vi "2 - Use the NI-DAQmx VIs (Original).vi"() -> ()   [LabVIEW 2012]
uses:
  <vilib>/DAQmx/read.llb/DAQmx Read (Analog 1D Wfm NChan NSamp).vi
  <vilib>/DAQmx/create/channels.llb/DAQmx Create Channel (AI-Temperature-Thermocouple).vi
  <resource>/objmgr/daqmx.rc
panel:
  out "Alarm Output":bool
  in  "Alarm Level":dbl=26.0
  out "Temperature":waveform(dbl)[](graph)
  in  "stop":bool
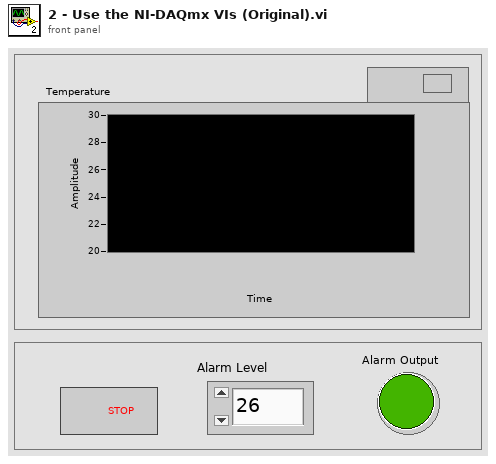
[diagram p1: front panel]
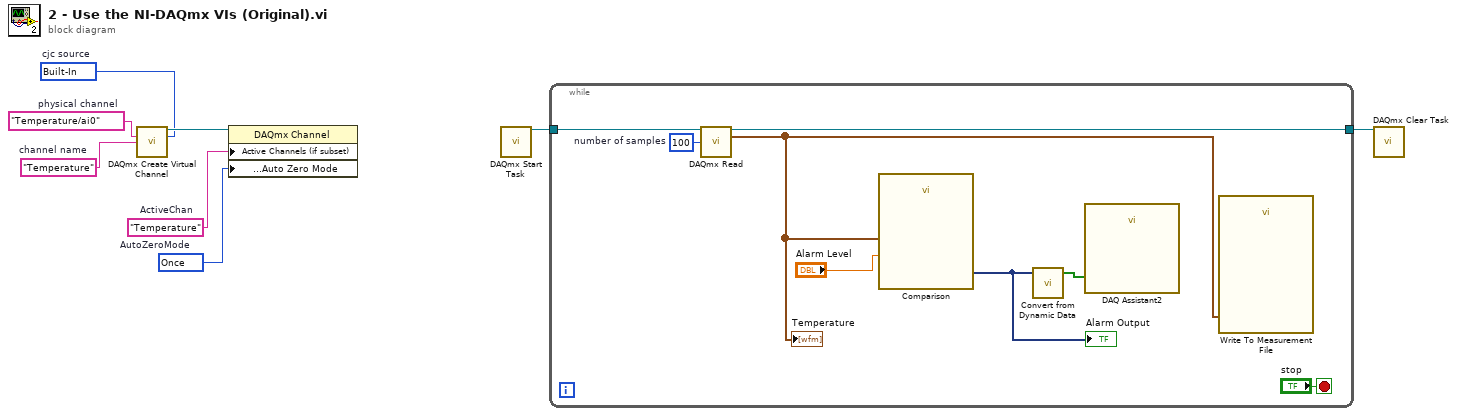
[diagram p0: block diagram]
diagram:
  w1 = tag "Temperature/ai0"  # physical channel
  w3 = 10200 items=["Built-In"=10200, "Constant Value"=10116, "Channel"=10113]  # cjc source
  w2 = 10244 items=["None"=10230, "Once"=10244, "Every Sample"=10164]  # AutoZeroMode
  w4 = "Temperature"  # ActiveChan
  w6 = "Temperature"  # channel name
  n1 = call-poly <vilib>:"DAQmx Create Virtual Channel.vi"("physical channels"=w1, "cjc source"=w3, "name to assign"=w6) -> ("task out"=w5:refnum<k21>)  [unwired: 11 in, 1 out]
  n2 = property class="DAQmx Channel"(reference=w5, "Active Channels (if subset)"=w4, "Analog Input:General Properties:Advanced:High Accuracy Settings:Auto Zero Mode"=w2) -> ()  [unwired: 1 in, 2 out]
  n3 = call <vilib>:"DAQmx Start Task.vi"() -> ("task out"=w8:refnum<k21>)  [unwired: 14 in, 1 out]
  n4 = while {
    tunnel: w8 -> [w12]
    tunnel: [w11] -> w7
    stop <- "stop" stop-if-true
    w9 = 100  # number of samples
    n5 = call-poly <vilib>:"DAQmx Read.vi"("task/channels in"=w12, "number of samples per channel"=w9) -> ("task out"=w11:refnum<k21>, "data"=w10:waveform(dbl)[])  [unwired: 11 in, 1 out]
    "Temperature" <- w10
    n6 = call "Comparison"("Operand 2"="Alarm Level", "Operand 1"=w10) -> ("Result"=w14:dynamicdata)  [unwired: 1 in, 8 out]
    "Alarm Output" <- w14
    n7 = call "Convert from Dynamic Data"("Dynamic Data Type"=w14) -> ("Array"=w13:bool[])  [unwired: 3 in]
    n8 = call "DAQ Assistant2"("data"=w13) -> ()  [unwired: 4 in, 15 out]
    n9 = call "Write To Measurement File"("Signals"=w10) -> ()  [unwired: 16 in, 3 out]
  }
  n10 = call <vilib>:"DAQmx Clear Task.vi"("task in"=w7) -> ()  [unwired: 14 in, 1 out]
